vi "Extended User Data.vi"(7 "Action":i32(ring) items=["Read Data", "Write Data", "Clear Data", "Clear ALL Data"], 8 "error in (no error)":errorcluster, 10 "User Data In":T1 {"Measurement Type" items=["DC Volts", "AC Volts", "DC Current", "AC Current", "2-Wire Resistance", "Frequency", "Temperature", "Capacitance", "Continuity", "Diode", "4-Wire Resistance"]; "344XX Mode" items=["34405A", "34450A"]}, 11 "VISA resource name in":refnum<visa-resource-name>) -> (0 "error out":errorcluster, 2 "User Data Out":T1 {"Measurement Type" items=["DC Volts", "AC Volts", "DC Current", "AC Current", "2-Wire Resistance", "Frequency", "Temperature", "Capacitance", "Continuity", "Diode", "4-Wire Resistance"]; "344XX Mode" items=["34405A", "34450A"]}, 3 "VISA resource name out":refnum<visa-resource-name>)   [LabVIEW 2020, in "Agilent 34405.lvlib"]
doc: "Performs an action on current VI settings (Measurment Type), such as write, read, clear and clear all."
uses:
  <instrlib>/Agilent 34405/Agilent 34405.lvlib
  <instrlib>/Agilent 34405/Private/Extended User Data.ctl
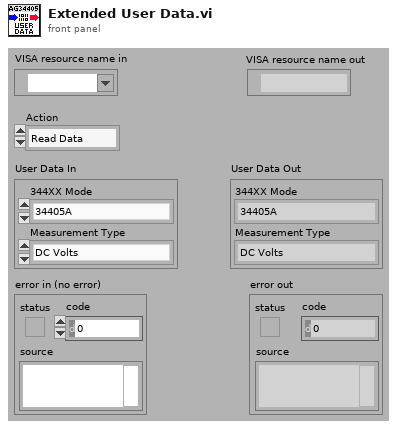
[diagram p1: front panel]
types:
  T1 = typedef "Agilent 34405.lvlib/Extended User Data.ctl" = cluster{"344XX Mode":u16, "Measurement Type":u16}
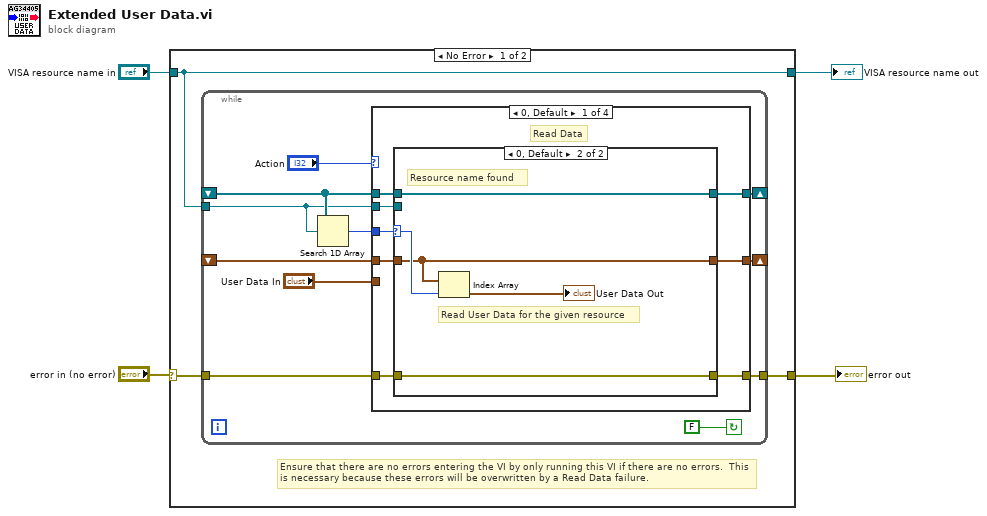
[diagram p0: block diagram]
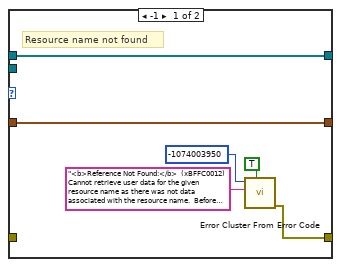
[diagram p2: hidden frame]
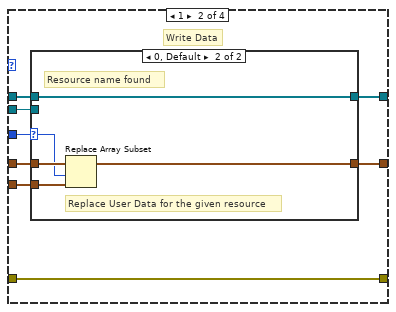
[diagram p3: hidden frame]
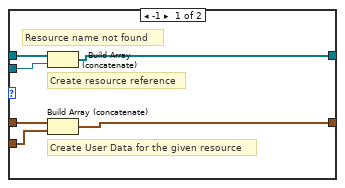
[diagram p4: hidden frame]
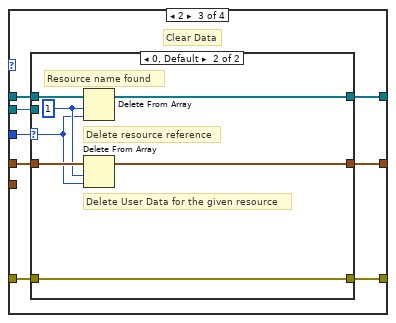
[diagram p5: hidden frame]
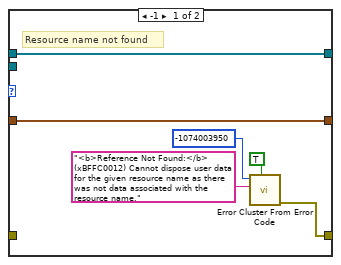
[diagram p6: hidden frame]
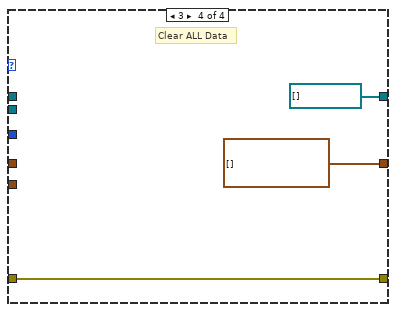
[diagram p7: hidden frame]
diagram:
  n1 = case shown="No Error" "error in (no error)" {
    selector: "error in (no error)" -> [w6 w82]
    tunnel: "VISA resource name in" -> [w5 w81]
    tunnel: [w7 w82] -> w3
    tunnel: [w5 w81] -> w4
    frame No Error {
      # "Ensure that there are no errors entering the VI by only running this VI if there are no errors.  This is necessary because these errors will be overwritten by a Read Data failure."
      n2 = while {
        shift-right: [w14] -> _
        shift-left: _ -> [w15]
        shift-right: [w17] -> _
        shift-left: _ -> [w18]
        tunnel: w5 -> [w13]
        tunnel: w6 -> [w11]
        tunnel: [w10] -> w7
        stop <- FALSE continue-if-true
        n3 = Search 1D Array(1D array=w15, element=w13) -> (index of element=w16:i32)  [unwired: 1 out]
        n4 = case shown="0, Default" "Action" {
          tunnel: w18 -> [w26 w45 w64 _]
          tunnel: [w25 w44 w63 T1[] []] -> w17
          tunnel: w16 -> [w24 w43 w62 _]
          tunnel: w15 -> [w23 w42 w61 _]
          tunnel: [w22 w41 w60 refnum<visa-resource-name>[] []] -> w14
          tunnel: w13 -> [w21 w40 w59 _]
          tunnel: w11 -> [w19 w39 w57 w79]
          tunnel: [w20 w39 w58 w79] -> w10
          tunnel: "User Data In" -> [_ w38 _ _]
          frame 0, Default {
            # "Read Data"
            n5 = case shown="0, Default" w24 {
              selector: w24 -> [_ w37]
              tunnel: [w31 w35] -> w25
              tunnel: w26 -> [w31 w35]
              tunnel: w23 -> [w32 w36]
              tunnel: [w32 w36] -> w22
              tunnel: w21 -> [_ _]
              tunnel: [w30 w34] -> w20
              tunnel: w19 -> [_ w34]
              frame -1 {
                # "Resource name not found"
                n6 = call <vilib>:"Error Cluster From Error Code.vi"("show call chain? (False)"=TRUE, "error message (\"\")"="<b>Reference Not Found:</b>  (xBFFC0012) Cannot retrieve user data for the given resource name as there was not data associated with the resource name.  Before you can read data, you need to write the user data using the Write Data action of this User Data VI. ", "error code (0)"=-1074003950 ("Code")) -> ("error out"=w30:errorcluster)  [unwired: 1 in, 5 out]
              }
              frame 0, Default {
                # "Read User Data for the given resource"
                # "Resource name found"
                n7 = Index Array(array=w35, index=w37) -> (element=→"User Data Out":T1)
              }
            }
          }
          frame 1 {
            # "Write Data"
            n8 = case shown="0, Default" w43 {
              selector: w43 -> [_ w54]
              tunnel: [w49 w56] -> w44
              tunnel: w45 -> [w50 w55]
              tunnel: w42 -> [w51 w53]
              tunnel: [w47 w53] -> w41
              tunnel: w40 -> [w48 _]
              tunnel: w38 -> [w46 w52]
              frame -1 {
                # "Create resource reference"
                # "Create User Data for the given resource"
                # "Resource name not found"
                n9 = Build Array (concatenate)(w51, w48) -> (w47:refnum<visa-resource-name>[])
                n10 = Build Array (concatenate)(w50, w46) -> (w49:T1[])
              }
              frame 0, Default {
                # "Replace User Data for the given resource"
                # "Resource name found"
                n11 = Replace Array Subset(array=w55, new element=w52, index=w54) -> (w56:T1[])
              }
            }
          }
          frame 2 {
            # "Clear Data"
            n12 = case shown="0, Default" w62 {
              selector: w62 -> [_ w71]
              tunnel: [w69 w77] -> w63
              tunnel: w64 -> [w69 w76]
              tunnel: w61 -> [w70 w74]
              tunnel: [w70 w73] -> w60
              tunnel: w59 -> [_ _]
              tunnel: [w68 w75] -> w58
              tunnel: w57 -> [_ w75]
              frame -1 {
                # "Resource name not found"
                n13 = call <vilib>:"Error Cluster From Error Code.vi"("show call chain? (False)"=TRUE, "error message (\"\")"="<b>Reference Not Found:</b>  (xBFFC0012) Cannot dispose user data for the given resource name as there was not data associated with the resource name.", "error code (0)"=-1074003950 ("Code")) -> ("error out"=w68:errorcluster)  [unwired: 1 in, 5 out]
              }
              frame 0, Default {
                w72 = 1 ("length")
                # "Delete resource reference"
                # "Delete User Data for the given resource"
                # "Resource name found"
                n14 = Delete From Array(array=w74, length=w72, index=w71) -> (array with subset deleted=w73:refnum<visa-resource-name>[])  [unwired: 1 out]
                n15 = Delete From Array(array=w76, length=w72, index=w71) -> (array with subset deleted=w77:T1[])  [unwired: 1 out]
              }
            }
          }
          frame 3 {
            # "Clear ALL Data"
          }
        }
      }
    }
    frame Error {
    }
  }
  "VISA resource name out" <- w4
  "error out" <- w3
